vi "Arrays With Enums.vi"(8 "Array Of Clusters With Enums 2":T4(array[cluster])=[{"Numeric"=1122.0, "Inner Cluster - Level 1"={"String"="Numeric Value 1122", "Boolean"=TRUE, "Enum"=enum."DDDD", "Numbers Enum"=enum."Three", "Text & Picture Control"=2513872035554745107, "Array"=[{"Numeric"=225.0, "String"="Number 225", "Text Ring"=4455, "Array Of Enums"=[enum."One", enum."Four", enum."Zero", enum."Four"], "Text Ring Control"=1}, {"Numeric"=1115.0, "String"="Value 1115", "Text Ring"=2233, "Array Of Enums"=[enum."Three", enum."Four", enum."Zero", enum."Three"], "Text Ring Control"=2}]}}, {"Numeric"=5.0, "Inner Cluster - Level 1"={"String"="FooBAR", "Boolean"=TRUE, "Enum"=enum."EEEE", "Numbers Enum"=enum."Five", "Text & Picture Control"=1722372036854595802, "Array"=[{"Numeric"=12345.0, "String"="Value 12345", "Text Ring"=4455, "Array Of Enums"=[enum."One", enum."Five", enum."Three", enum."Four"], "Text Ring Control"=1}, {"Numeric"=1122.0, "String"="aaaaaa", "Text Ring"=4455, "Array Of Enums"=[enum."One", enum."Four", enum."Five"], "Text Ring Control"=2}]}}] {"Inner Cluster - Level 1"."Text & Picture Control" items=["Home Sweet Home!"=9223372036854775807, "Zero In Chinese"=0, "Another Piece Of The Puzzle"=9000000006854770000, "Hmmm ????"=5729325037854735917, "The Connector Pane"=7213312035854725405, "Look At The Fish"=2513872035554745107, "Its A Turtle!"=1722372036854595802]; "Inner Cluster - Level 1"."Array"."Text Ring Control" items=["Text Value 0", "Text Value 1", "Text Value 2", "Text Value 3", "Text Value 5", "Text Value 6"]; "Inner Cluster - Level 1"."Array"."Text Ring" items=["Text Ring Value 1"=111, "Text Ring Value 2"=2233, "Text Ring Value 3"=4455, "Text Ring Value 4"=5566, "Text Ring Value 5"=7788]}, 9 "Array Of Clusters With Enums":T5(array[cluster])=[{"Numeric"=11.0, "Inner Cluster - Level 1"={"String"="Numeric Value 111", "Boolean"=TRUE, "Enum"=enum."EEEE", "Numbers Enum"=enum."Two", "Text Ring Control"=0, "Cluster"={"Numeric"=345.0, "String"="Value 345", "Text Ring"=5566}}}, {"Numeric"=4561.0, "Inner Cluster - Level 1"={"String"="Value 4561", "Boolean"=FALSE, "Enum"=enum."BBB", "Numbers Enum"=enum."Four", "Text Ring Control"=0, "Cluster"={"Numeric"=5577.0, "String"="Value 5577", "Text Ring"=111}}}] {"Inner Cluster - Level 1"."Text Ring Control" items=["Text Value 0", "Text Value 1", "Text Value 2", "Text Value 3", "Text Value 5", "Text Value 6"]; "Inner Cluster - Level 1"."Cluster"."Text Ring" items=["Text Ring Value 1"=111, "Text Ring Value 2"=2233, "Text Ring Value 3"=4455, "Text Ring Value 4"=5566, "Text Ring Value 5"=7788]}, 10 "Array Of Text Ring":T1[](array[typedef])=[4, 5, 1] items=["Text Value 0", "Text Value 1", "Text Value 2", "Text Value 3", "Text Value 5", "Text Value 6"], 11 "Array Of Enums":T2[](array[typedef])=[enum."Three", enum."Five", enum."One", enum."Two"]) -> ()   [LabVIEW 2012]
uses:
  EnumTypeDefControl.ctl
  TextRingTypeDefControl.ctl
  Text&PictTypeDefControl.ctl
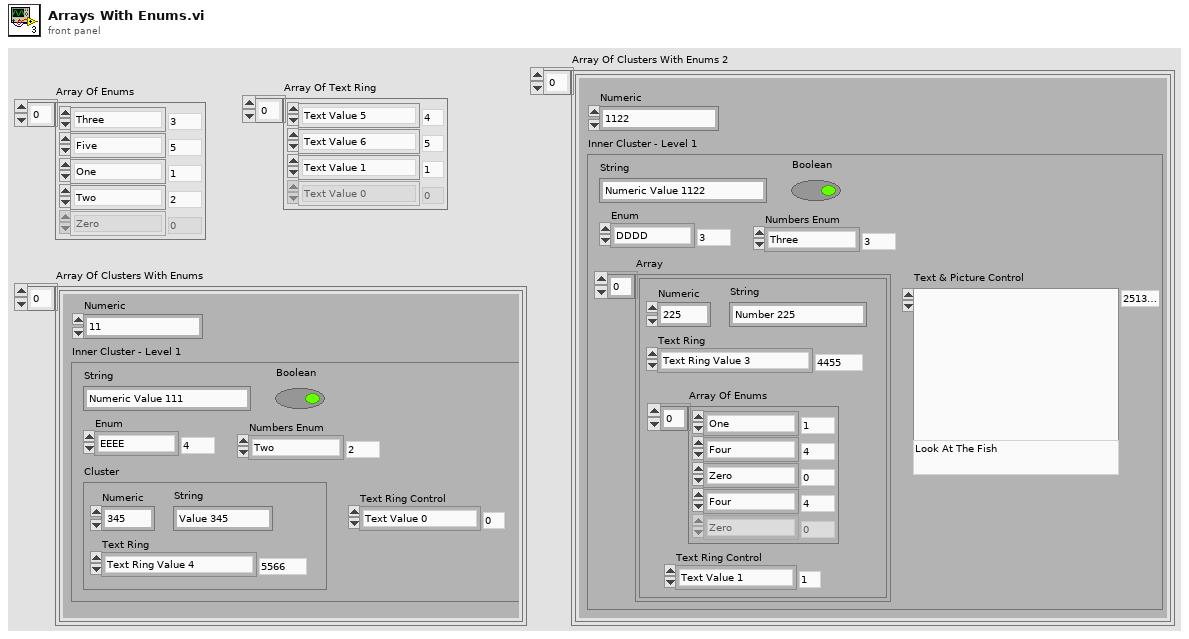
[diagram p1: front panel]
types:
  T1 = typedef "TextRingTypeDefControl.ctl" = u16
  T2 = typedef "EnumTypeDefControl.ctl" = enum8{"Zero", "One", "Two", "Three", "Four", "Five"}
  T3 = typedef "Text&PictTypeDefControl.ctl" = i64
  T4 = cluster{"Numeric":dbl, "Inner Cluster - Level 1":cluster{"String":string, "Boolean":bool, "Enum":enum16{"AAA", "BBB", "CCCC", "DDDD", "EEEE"}, "Numbers Enum":T2, "Text & Picture Control":T3, "Array":cluster{"Numeric":dbl, "String":string, "Text Ring":u16, "Array Of Enums":T2[], "Text Ring Control":T1}[]}}[]
  T5 = cluster{"Numeric":dbl, "Inner Cluster - Level 1":cluster{"String":string, "Boolean":bool, "Enum":enum16{"AAA", "BBB", "CCCC", "DDDD", "EEEE"}, "Numbers Enum":T2, "Text Ring Control":T1, "Cluster":cluster{"Numeric":dbl, "String":string, "Text Ring":u16}}}[]
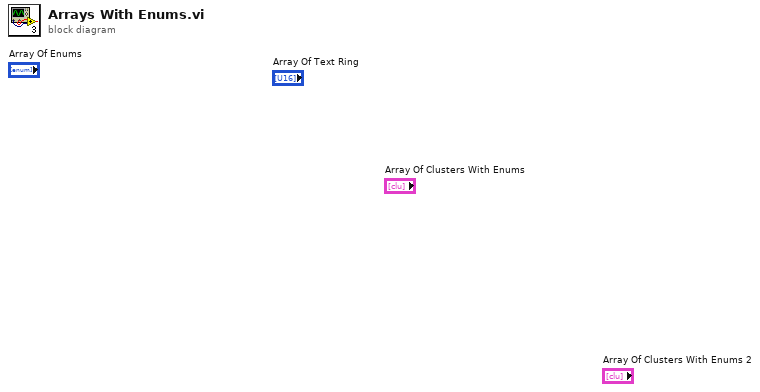
[diagram p0: block diagram]
diagram:
